vi "Init Events.vi"(8 "error in (no error)":errorcluster, 11 "GVIWebProcessorApp in":refnum<class "GVIWebProcessorApp.lvclass">) -> (0 "error out":errorcluster, 3 "GVIWebProcessorApp out":refnum<class "GVIWebProcessorApp.lvclass">)   [LabVIEW 2020, in "PicoG-Processor.lvlib" / "GVIWebProcessorApp.lvclass"]
uses:
  GVIWebProcessorApp.lvclass
  Close Event Data.ctl
  Refresh Event Data.ctl
  Set Collapsed UI Event.ctl
  WebProjectWatcher/Web Build.ctl
  GVIWebProcessorApp.lvclass/GVIWebProcessorApp.ctl
  WebProjectWatcher/WebProjectWatcher.lvclass
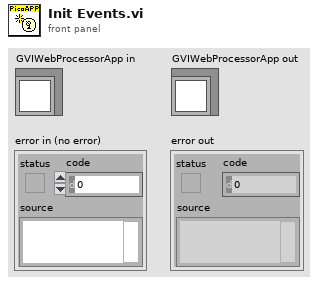
[diagram p1: front panel]
types:
  T1 = typedef "PicoG-Processor.lvlib/WebProjectWatcher.lvclass/Web Build.ctl" = cluster{"Name":string, "Path":path, "Last Update":dbl}
  T2 = typedef "PicoG-Processor.lvlib/GVIWebProcessorApp.lvclass/Set Collapsed UI Event.ctl" = bool
  T3 = typedef "PicoG-Processor.lvlib/GVIWebProcessorApp.lvclass/Refresh Event Data.ctl" = bool
  T4 = typedef "PicoG-Processor.lvlib/GVIWebProcessorApp.lvclass/Close Event Data.ctl" = bool
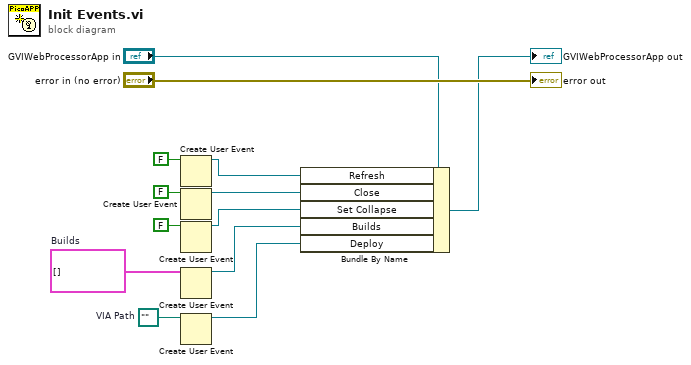
[diagram p0: block diagram]
diagram:
  w2 = path ""  # VIA Path
  w4 = T1[] []  # Builds
  n1 = Create User Event(user event datatype=T3 FALSE ("Refresh")) -> (user event=w7:refnum<user-event>)  [unwired: 1 in, 1 out]
  n2 = Create User Event(user event datatype=T4 FALSE ("Close")) -> (user event=w8:refnum<user-event>)  [unwired: 1 in, 1 out]
  n3 = Create User Event(user event datatype=T2 FALSE ("Collapsed")) -> (user event=w5:refnum<user-event>)  [unwired: 1 in, 1 out]
  n4 = Create User Event(user event datatype=w4) -> (user event=w3:refnum<user-event>)  [unwired: 1 in, 1 out]
  n5 = Create User Event(user event datatype=w2) -> (user event=w1:refnum<user-event>)  [unwired: 1 in, 1 out]
  n6 = Bundle By Name(cluster="GVIWebProcessorApp in", "Refresh"=w7, "Close"=w8, "Set Collapse"=w5, "Builds"=w3, "Deploy"=w1) -> (→"GVIWebProcessorApp out":refnum<class "GVIWebProcessorApp.lvclass">)
  "error out" <- "error in (no error)"
